vi "QuitSubSystem.vi"(6 "InitFlags":T1 items=["NONE"=0, "SDL_INIT_AUDIO"=16, "SDL_INIT_VIDEO"=32, "SDL_INIT_JOYSTICK"=512, "SDL_INIT_HAPTIC"=4096, "SDL_INIT_GAMEPAD"=8192, "SDL_INIT_EVENTS"=16384, "SDL_INIT_SENSOR"=32768, "SDL_INIT_CAMER"=65536], 8 "No Error":errorcluster) -> (0 "error out":errorcluster)   [LabVIEW 2026, in "SDL3.lvlib" / "Init.lvlib"]
doc: "<B>Summary</B>\nShut down specific SDL subsystems.\n\n<B>Remarks</B>\nYou still need to call <B>SDL_Quit()</B> even if you close all open subsystems with <B>SDL_QuitSubSystem()</B>."
uses:
  Init.lvlib
  InitFlags--ring.ctl
  Lib/SDL3.dll
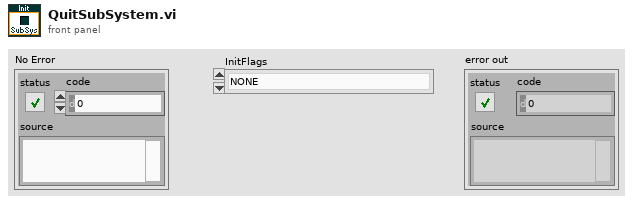
[diagram p1: front panel]
types:
  T1 = typedef "SDL3.lvlib/Init.lvlib/InitFlags--ring.ctl" = u32
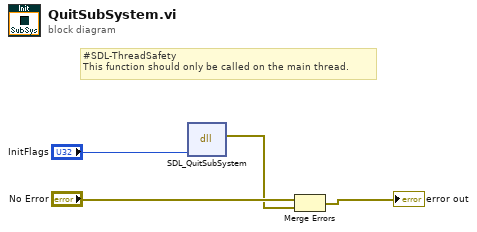
[diagram p0: block diagram]
diagram:
  # "#SDL-ThreadSafety\nThis function should only be called on the main thread."
  n1 = dll-call lib="C:/Users/saukko/Dev/LV-SDL3/Sources/SDL3/Lib/SDL3.*" fn="SDL_QuitSubSystem"("flags"="InitFlags") -> (error out=w1:errorcluster)  [unwired: 5 in, 1 out]
  n2 = Merge Errors("No Error", w1) -> (→"error out":errorcluster)
